vi "IdentificarObjeto.vi"(10 "Error in":errorcluster, 11 "Session In":T1) -> (1 "Objeto Detectado":string, 2 "Image":T2(plugin-control))   [LabVIEW 2020]
doc: "Este VI implementa el algoritmo de identificación para la imagen adquirida por la cámara. Se toma el promedio de 5 imágenes consecutivas y se mandar a llamar al subVI Detección_ROI. Despúes, se normaliza la imagen a un tamaño de 400x250 pixeles y se convierte en un vector de 1x(400x250x3) que contiene la información de los 3 canales RGB. El vecotr se normaliza y después, se recupera la base y puntos de cada objeto en la base, se calcula el punto que ocupa en el espacio k-dimensional de cada objeto el vector obtenido, y después se calcúla la distancia mínima de todos los puntos en los espacios. Posteriormente, se obtiene estas distancias mínimas asociadas a cada objeto y se declara que el vector es el objeto con distancia mínima."
uses:
  <vilib>/userdefined/High Color/IMAQdx.ctl
  <vilib>/Analysis/baseanly.llb/Mean (DBL).vi
  Global_archivobasedatos.vi
  <vilib>/addons/database/Connection.llb/DB Tools Open Connec (Path).vi
  <vilib>/addons/database/Connection.llb/Conn Execute.vi
  <vilib>/addons/database/Recordset.llb/Rec Fetch Recordset Data (R).vi
  <vilib>/Analysis/BLAS.llb/dgemv - General Matrix-Vector Product (DBL).vi
  <vilib>/addons/database/Recordset.llb/Rec Destroy - Connection.vi
  <vilib>/addons/database/_DB Variant To Data/Database Variant To Data.xnode
  <vilib>/addons/database/NI_Database_API.lvlib
  <vilib>/vision/driver/NI_Vision_Acquisition_Software.lvlib
  <vilib>/vision/NI_Vision_Development_Module.lvlib
  <vilib>/Analysis/NI_AALBLAS.lvlib
  <vilib>/Analysis/NI_AALBase.lvlib
panel:
  out "Errores":dbl[](array[numeric])
  out "Distancias mínimas":dbl[](array[numeric])
  out "Lista de objetos":string[](array[string])
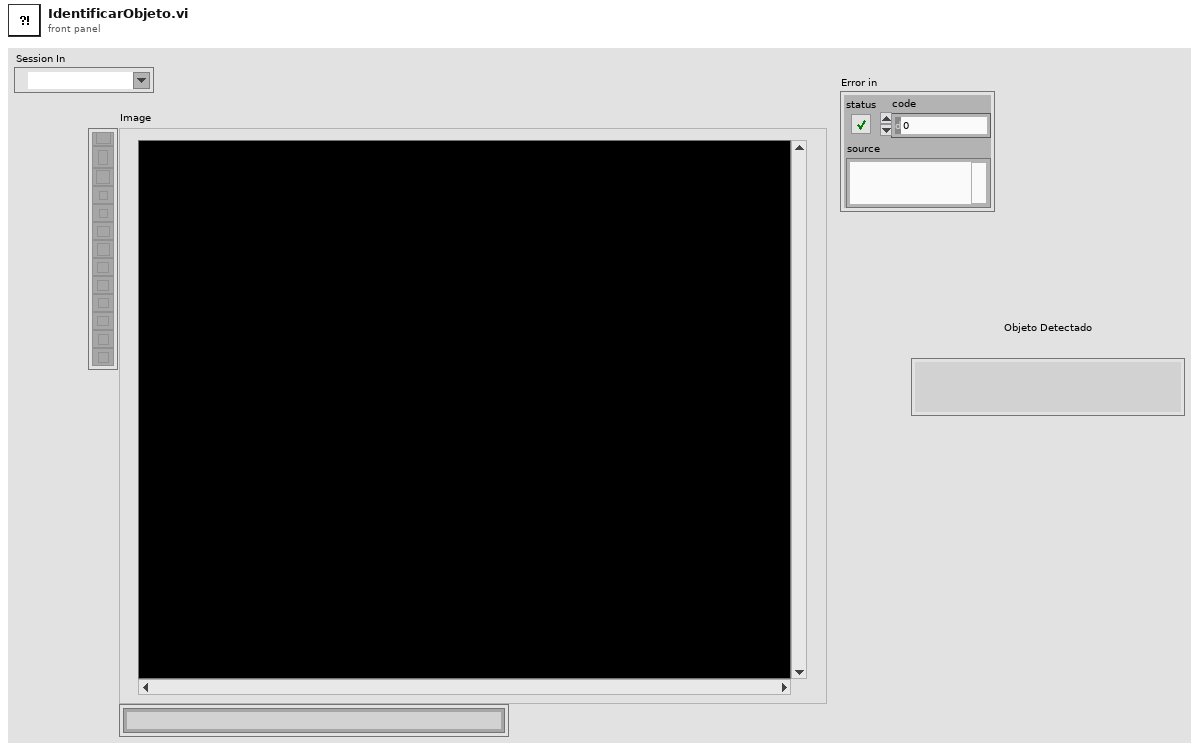
[diagram p1: front panel]
types:
  T1 = typedef "IMAQdx.ctl" = refnum<k21>
  T2 = typedef "IMAQ Image.ctl" = refnum<image>
  T3 = typedef "Image Type" = u32
  T4 = typedef "NI_Database_API.lvlib/Conn ObjectReference.ctl" = refnum<k1>
  T5 = typedef "NI_Database_API.lvlib/Rec ObjectReference.ctl" = refnum<k1>
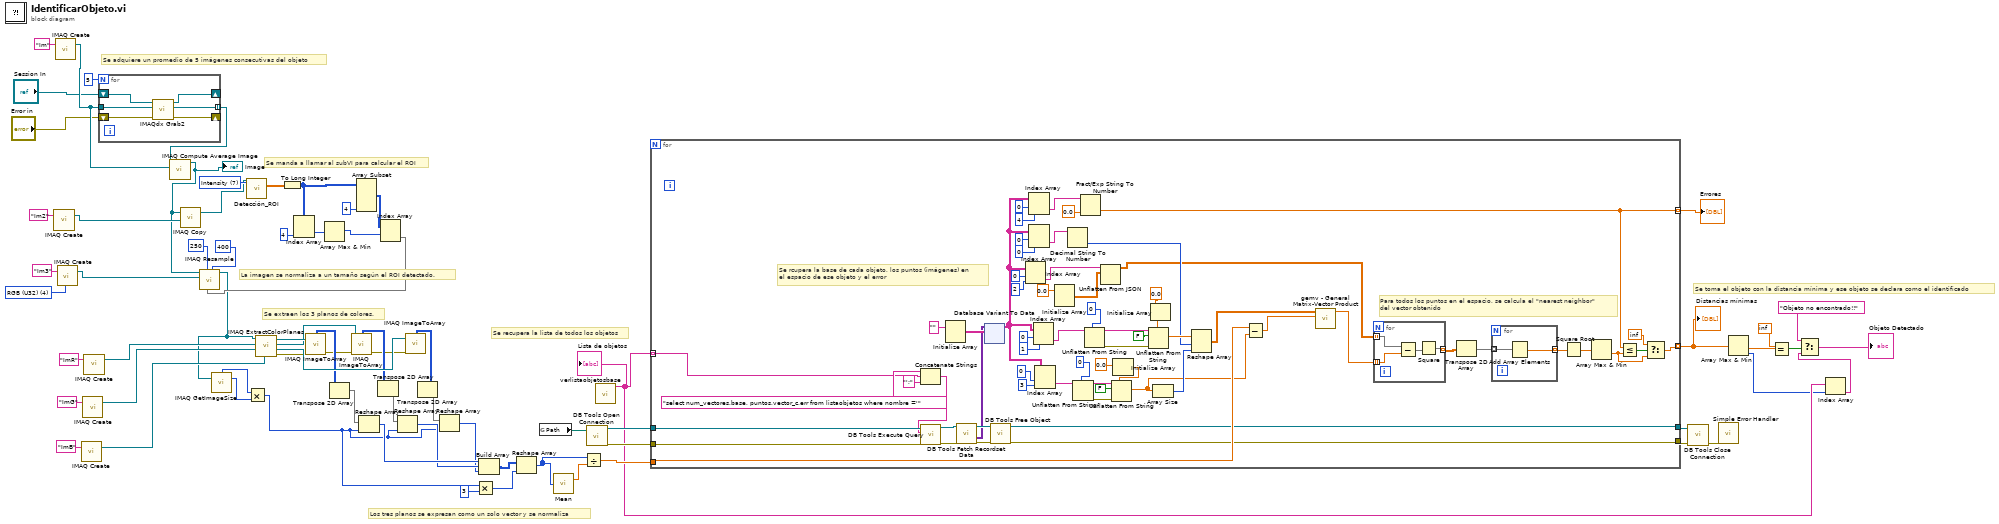
[diagram p0: block diagram]
diagram:
  w34 = 7 items=["Red", "Green", "Blue", "Hue", "Saturation", "Luminance", "Value", "Intensity"] ("Color Plane (Color Plane Extraction 1)")
  w35 = T3 4 items=["Grayscale (U8)", "Grayscale (I16)", "Grayscale (SGL)", "Complex (CSG)", "RGB (U32)", "HSL (U32)", "RGB (U64)", "Grayscale (U16)"] ("Image Type")
  # "Se toma el objeto con la distancia mínima y ese objeto se declara como el identificado"
  # "Se recupera la lista de todos los objetos"
  # "Los tres planos se expresan como un solo vector y se normaliza"
  # "Se extraen los 3 planos de colores."
  # "La imagen se normaliza a un tamaño según el ROI detectado."
  # "Se manda a llamar al subVI para calcular el ROI"
  # "Se adquiere un promedio de 5 imágenes consecutivas del objeto"
  n1 = call "IMAQ Create"("Image Name"="Im2") -> ("New Image"=w21:T2)  [unwired: 4 in, 1 out]
  n2 = call "IMAQ Create"("Image Name"="Im") -> ("New Image"=w15:T2)  [unwired: 4 in, 1 out]
  n3 = call "IMAQ Create"("Image Name"="Im3", "Image Type"=w35) -> ("New Image"=w22:T2)  [unwired: 3 in, 1 out]
  n4 = call "IMAQ Create"("Image Name"="ImB") -> ("New Image"=w63:T2)  [unwired: 4 in, 1 out]
  n5 = call "IMAQ Create"("Image Name"="ImG") -> ("New Image"=w64:T2)  [unwired: 4 in, 1 out]
  n6 = call "IMAQ Create"("Image Name"="ImR") -> ("New Image"=w65:T2)  [unwired: 4 in, 1 out]
  n7 = for {
    N: 5 -> [_]
    tunnel: w15 -> [w75]
    shift-right: [w74] -> _
    shift-left: "Session In" -> [w77]
    shift-right: [w73] -> _
    shift-left: "Error in" -> [w76]
    tunnel: [w72] -> w17 mode=indexing
    n8 = call <vilib>:"IMAQdx Grab2.vi"("error in"=w76, "Image In"=w75, "Session In"=w77) -> ("error out"=w73:errorcluster, "Image Out"=w72:T2, "Session Out"=w74:T1)  [unwired: 5 in, 1 out]
  }
  n9 = call "IMAQ Compute Average Image"("Image Dst"=w15, "Images"=w17) -> ("Image Dst Out"=w16:T2)  [unwired: 8 in, 1 out]
  "Image" <- w16
  n10 = call "IMAQ Copy"("Image Dst"=w21, "Image Src"=w16) -> ("Image Dst Out"=w26:T2)  [unwired: 4 in, 1 out]
  n11 = call "Detección_ROI.vi"("Image In"=w26, "Color Plane (Color Plane Extraction 1)"=w34) -> ("Particle Measurements (Pixels) (Particle Analysis 1)"=w33:dbl[][])  [unwired: 21 in, 4 out]
  n12 = To Long Integer(number=w33) -> (32bit integer=w31:i32[][])
  n13 = Index Array(array=w31, index (col)=4 ("disabled index (col)")) -> (element=w29:i32[])  [unwired: 1 in]
  n14 = Array Max & Min(array=w29) -> (max index (indices)=w27:i32)  [unwired: 3 out]
  n15 = Array Subset(array=w31, length (col)=4 ("length")) -> (w28:i32[][])  [unwired: 3 in]
  n16 = Index Array(array=w28, index (row)=w27) -> (element=w23:i32[])  [unwired: 1 in]
  n17 = call "IMAQ Resample"("X Resolution"=400 ("Y Resolution"), "Optional Rectangle"=w23, "Y Resolution"=250, "Image Dst"=w22, "Image Src"=w16) -> ("Image Dst Out"=w20:T2)  [unwired: 5 in, 1 out]
  n18 = call "IMAQ GetImageSize"("Image"=w20) -> ("Y Resolution"=w54:i32, "X Resolution"=w53:i32)  [unwired: 3 in, 1 out]
  n19 = Multiply(x=w53, y=w54) -> (x*y=w49:i32)
  n20 = call "IMAQ ExtractColorPlanes"("Blue or Luma or Val or Inten Plane"=w63, "Green or Sat Plane"=w64, "Red or Hue Plane"=w65, "Image Src"=w20) -> ("error out"=w42:errorcluster, "Blue or Luma or Val or Inten Plane out"=w62:T2, "Green or Sat Plane out"=w43:T2, "Red or Hue Plane out"=w61:T2)  [unwired: 4 in]
  n21 = call "IMAQ ImageToArray"("error in (no error)"=w42, "Image"=w61) -> ("error out"=w41:errorcluster, "Image Pixels (U8)"=w60:u8[][])  [unwired: 2 in, 3 out]
  n22 = Transpose 2D Array(2D array=w60) -> (transposed array=w57:u8[][])
  n23 = call "IMAQ ImageToArray"("error in (no error)"=w41, "Image"=w43) -> ("error out"=w40:errorcluster, "Image Pixels (U8)"=w59:u8[][])  [unwired: 2 in, 3 out]
  n24 = Reshape Array(w57, w49) -> (w52:u8[])
  n25 = Transpose 2D Array(2D array=w59) -> (transposed array=w56:u8[][])
  n26 = Reshape Array(w56, w49) -> (w51:u8[])
  n27 = call "IMAQ ImageToArray"("error in (no error)"=w40, "Image"=w62) -> ("Image Pixels (U8)"=w58:u8[][])  [unwired: 2 in, 4 out]
  n28 = Transpose 2D Array(2D array=w58) -> (transposed array=w55:u8[][])
  n29 = Reshape Array(w55, w49) -> (w50:u8[])
  n30 = Multiply(x=w49, y=3) -> (x*y=w47:i32)
  n31 = Build Array(w52, w51, w50) -> (w46:u8[][])
  n32 = Reshape Array(w46, w47) -> (w39:u8[])
  n33 = global read "Global_archivobasedatos.vi" "Path"() -> (w14:path)
  n34 = call-poly <vilib>:"Mean.vi"("X"=w39) -> ("mean"=w38:dbl)  [unwired: 1 out]
  n35 = Divide(x=w39, y=w38) -> (x/y=w45:dbl[])
  n36 = call-poly <vilib>:"DB Tools Open Connection.vi"("connection information"=w14) -> ("error out"=w71:errorcluster, "connection reference"=w70:T4)  [unwired: 7 in]
  n37 = call "verlistaobjetosbase.vi"() -> ("lista_objetos"=w19:string[])  [unwired: 11 in]
  "Lista de objetos" <- w19
  n38 = for {
    tunnel: w71 -> [w135]
    tunnel: w70 -> [w134]
    tunnel: w19 -> [w120] mode=indexing
    tunnel: w45 -> [w111]
    tunnel: [w105] -> w12
    tunnel: [w106] -> w13
    tunnel: [w79] -> w11 mode=indexing
    tunnel: [w78] -> w3 mode=indexing
    # "Para todos los puntos en el espacio, se calcula el \"nearest neighbor\" \ndel vector obtenido"
    # "Se rcupera la base de cada objeto, los puntos (imágenes) en \nel espacio de ese objeto y el error"
    n39 = Concatenate Strings("select num_vectores,base, puntos,vector_c,err from listaobjetos where nombre ='", w120, "';" ("string")) -> (w131:string)
    n40 = call-poly <vilib>:"DB Tools Execute Query.vi"("error in (no error)"=w135, "SQL query"=w131, "connection reference"=w134) -> ("error out"=w137:errorcluster, "recordset reference"=w136:T5)  [unwired: 5 in]
    n41 = Initialize Array("") -> (w141:string[][])  [unwired: 2 in]
    n42 = call-poly <vilib>:"DB Tools Fetch Recordset Data.vi"("error in (no error)"=w137, "recordset reference"=w136) -> ("error out"=w139:errorcluster, "recordset data"=w121:variant[][], "recordset reference out"=w138:T5)  [unwired: 3 in]
    n43 = xnode "Database Variant To Data"("database variant"=w121, "type"=w141) -> ("data"=w87:string[][])  [unwired: 1 in, 1 out]
    n44 = call-poly <vilib>:"DB Tools Free Object.vi"("error in (no error)"=w139, "recordset reference"=w138) -> ("error out"=w105:errorcluster, "connection reference"=w106:T4)  [unwired: 8 in]
    n45 = Index Array(array=w87, index (row)=0 ("disabled index (row)"), index (col)=2 ("index (row)")) -> (element=w128:string)
    n46 = Index Array(array=w87, index (row)=0, index (col)=4 ("disabled index (col)")) -> (element=w84:string)
    n47 = Index Array(array=w87, index (row)=0, index (col)=0 ("disabled index (col)")) -> (element=w96:string)
    n48 = Index Array(array=w87, index (row)=0, index (col)=1) -> (element=w100:string)
    n49 = Index Array(array=w87, index (row)=0, index (col)=3) -> (element=w119:string)
    n50 = Initialize Array(0.0 ("element")) -> (w126:dbl[][])  [unwired: 2 in]
    n51 = Decimal String To Number(string=w96) -> (number=w92:i32)  [unwired: 2 in, 1 out]
    n52 = Unflatten From String(type=0, binary string=w119) -> (rest of the binary string=w116:string, error out=w117:errorcluster)  [unwired: 3 in, 1 out]
    n53 = Fract/Exp String To Number(string=w84, default (0 dbl)=0.0 ("default (0 DBL)")) -> (number=w78:dbl)  [unwired: 2 in, 1 out]
    n54 = Unflatten From String(type=0, binary string=w100) -> (rest of the binary string=w103:string, error out=w102:errorcluster)  [unwired: 3 in, 1 out]
    n55 = Unflatten From JSON(JSON string=w128, type and defaults=w126) -> (value=w90:dbl[][])  [unwired: 5 in, 1 out]
    n56 = Initialize Array(0.0 ("element")) -> (w113:dbl[])  [unwired: 1 in]
    n57 = Unflatten From String(type=w113, binary string=w116, data includes array or string size? (T)=FALSE, error in (no error)=w117) -> (value=w89:dbl[])  [unwired: 1 in, 2 out]
    n58 = Initialize Array(0.0 ("element")) -> (w99:dbl[])  [unwired: 1 in]
    n59 = Unflatten From String(type=w99, binary string=w103, data includes array or string size? (T)=FALSE, error in (no error)=w102) -> (value=w94:dbl[])  [unwired: 1 in, 2 out]
    n60 = Array Size(array=w89) -> (size(s)=w93:i32)
    n61 = Reshape Array(w94, w92, w93) -> (w88:dbl[][])
    n62 = Subtract(x=w111, y=w89) -> (x-y=w112:dbl[])
    n63 = call-poly <vilib>:"gemv - General Matrix-Vector Product.vi"("x"=w112, "A"=w88) -> ("dgemv"=w91:dbl[])  [unwired: 8 in, 1 out]
    n64 = for {
      tunnel: w90 -> [w147] mode=indexing
      tunnel: w91 -> [w146] mode=indexing
      tunnel: [w144] -> w110 mode=indexing
      n65 = Subtract(x=w147, y=w146) -> (x-y=w145:dbl[])
      n66 = Square(x=w145) -> (x^2=w144:dbl[])
    }
    n67 = Transpose 2D Array(2D array=w110) -> (transposed array=w109:dbl[][])
    n68 = for {
      tunnel: w109 -> [w143] mode=indexing
      tunnel: [w142] -> w108 mode=indexing
      n69 = Add Array Elements(numeric array=w143) -> (sum=w142:dbl)
    }
    n70 = Square Root(x=w108) -> (sqrt(x)=w107:dbl[])
    n71 = Array Max & Min(array=w107) -> (min value=w80:dbl)  [unwired: 3 out]
    n72 = Less Or Equal?(x=w78, y=w80) -> (x <= y?=w82:bool)
    n73 = Select(t=inf, s=w82, f=w80) -> (s? t:f=w79:dbl)
  }
  "Distancias mínimas" <- w11
  "Errores" <- w3
  n74 = call <vilib>:"DB Tools Close Connection.vi"("error in (no error)"=w12, "connection reference"=w13) -> ("error out"=w44:errorcluster)  [unwired: 5 in]
  n75 = call <vilib>:"Simple Error Handler.vi"("error in (no error)"=w44) -> ()  [unwired: 4 in, 5 out]
  n76 = Array Max & Min(array=w11) -> (min value=w10:dbl, min index (indices)=w5:i32)  [unwired: 2 out]
  n77 = Equal?(x=inf, y=w10) -> (x = y?=w8:bool)
  n78 = Index Array(array=w19, index=w5) -> (element=w4:string)
  n79 = Select(t="Objeto no encontrado!!", s=w8, f=w4) -> (s? t:f=→"Objeto Detectado":string)
